vi "Toggle.vi"(1 "Input":bool) -> (0 "Toggled Output":bool)   [LabVIEW 2016]
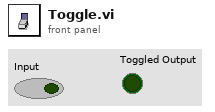
[diagram p1: front panel]
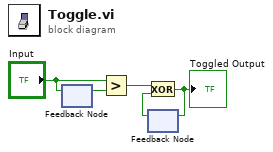
[diagram p0: block diagram]
diagram:
  n1 = feedback #1() -> (w1:bool)  [unwired: 1 in]
  n2 = feedback-in #1("Input") -> ()
  n3 = Greater?(x="Input", y=w1) -> (0:w2:bool)
  n4 = feedback #2() -> (w3:bool)  [unwired: 1 in]
  n5 = Exclusive Or(1:w3, 2:w2) -> (0:w4:bool)
  "Toggled Output" <- w4
  n6 = feedback-in #2(w4) -> ()
